vi "Rearrange Datagridview data.vi"(9 "Variables Data":string[][](array[string]), 10 "Device Type":string, 11 "Devicetype\n Variables":string[](array[string])) -> (3 "Array":T1(array[cluster]))   [LabVIEW 2020]
uses:
  <userlib>/_OpenG.lib/array/array.llb/Filter 1D Array (String)__ogtk.vi
  <userlib>/_OpenG.lib/array/array.llb/Delete Elements from 2D Array (String)__ogtk.vi
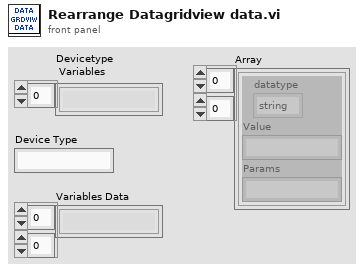
[diagram p1: front panel]
types:
  T1 = cluster{"datatype":enum16{"string", "image", "check", "numeric", "timestamp", "button", "combo", "link"}, "Value":string, "Params":string}[][]
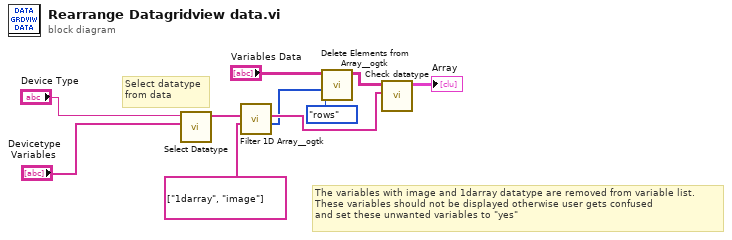
[diagram p0: block diagram]
diagram:
  # "The variables with image and 1darray datatype are removed from variable list.\nThese variables should not be displayed otherwise user gets confused \nand set these unwanted variables to \"yes\""
  # "Select datatype \nfrom data"
  n1 = call "Select Datatype.vi"("data"="Devicetype\n Variables", "Devicetype"="Device Type") -> ("Datatype"=w4:string[])  [unwired: 9 in]
  n2 = call-poly <userlib>:"Filter 1D Array__ogtk.vi"("items to filter"=string[] ["1darray", "image"], "array"=w4) -> ("filtered item indices"=w7:i32[], "filtered array"=w10:string[])  [unwired: 4 in]
  n3 = call-poly <userlib>:"Delete Elements from Array__ogtk.vi"("delete (rows or columns)"=enum16{"rows", "columns"}."rows", "indices"=w7, "array"="Variables Data") -> ("array w/ subset deleted"=w9:string[][])  [unwired: 7 in, 1 out]
  n4 = call "Check datatype.vi"("Datatype"=w10, "Data Array"=w9) -> ("Array"=→"Array":T1)  [unwired: 9 in]
